vi "Apply force DS345 TDC001 soft tw.vi"(4 "Moving parameters":T2={"Velocity (mm/s)"=0.5, "Abs position (mm)"=0.0, "Lasting time (s)"=20.0}, 5 "Lasting time (s)":dbl=10.0, 6 "TDC001 motor Serial":i32=83858441, 7 "Apply force":bool, 8 "Cluster":T1={"Osc. Amp. (V)"=0.06, "Osc. Freq. (Hz)"=1200.0} {"Osc. Freq. (Hz)" min=0.001 max=250000.0 step=0.001 format="%.3f"; "Osc. Amp. (V)" min=0.0 max=10.0 step=0.001 format="%.3f"}, 9 "Default setting (DS345)":T1={"Osc. Amp. (V)"=0.01, "Osc. Freq. (Hz)"=1000.0} {"Osc. Freq. (Hz)" min=0.001 max=250000.0 step=0.001 format="%.3f"; "Osc. Amp. (V)" min=0.0 max=0.1 step=0.001 format="%.3f"}, 10 "SRS DS345 GPIB address":string="0:18") -> ()   [LabVIEW 2015]
panel:
  out "Working":bool
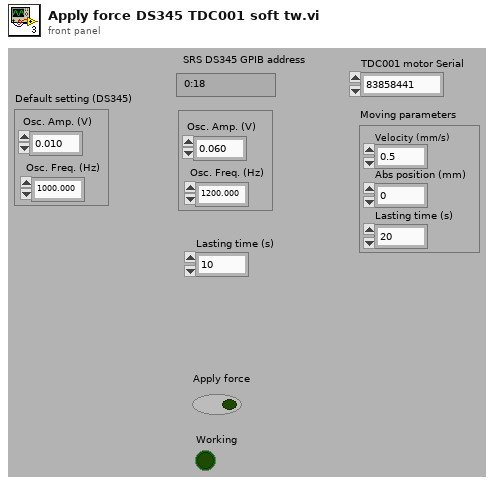
[diagram p1: front panel]
types:
  T1 = cluster{"Osc. Amp. (V)":dbl, "Osc. Freq. (Hz)":dbl}
  T2 = cluster{"Velocity (mm/s)":dbl, "Abs position (mm)":dbl, "Lasting time (s)":dbl}
  T3 = cluster{"Velocity (mm/s)":dbl, dbl, "Lasting time (s)":dbl}
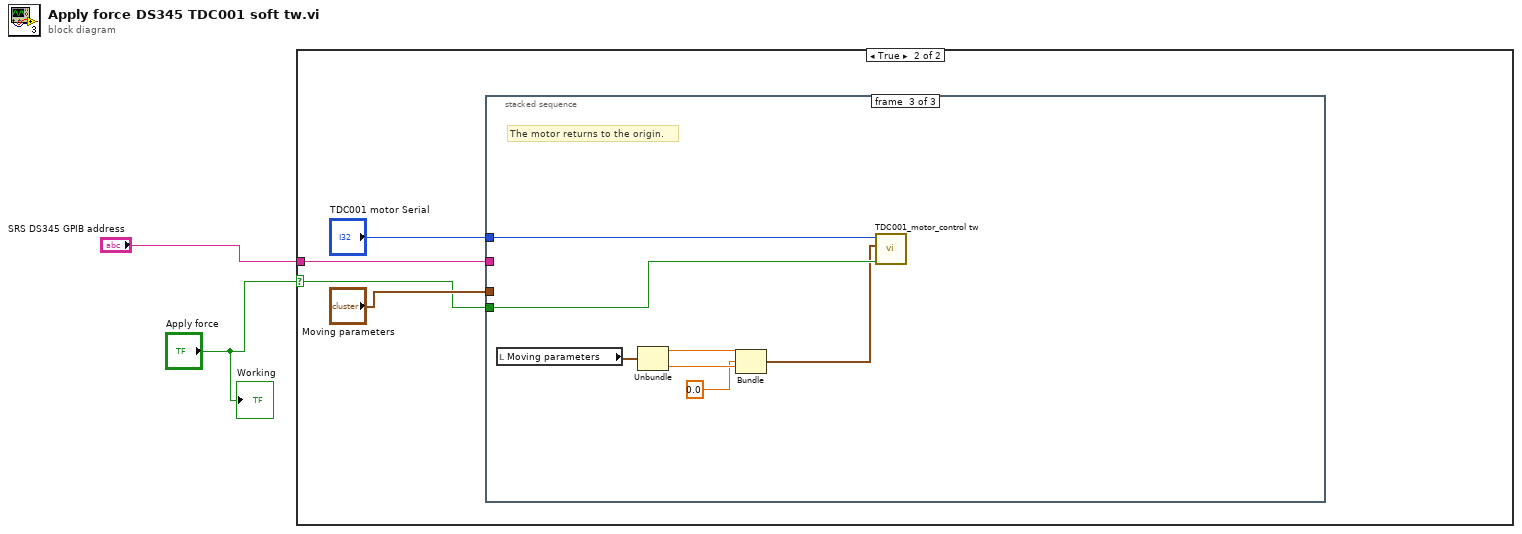
[diagram p0: block diagram]
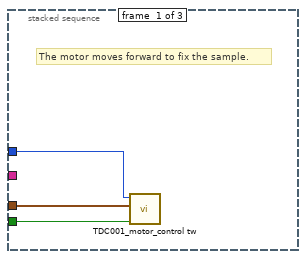
[diagram p3: hidden frame]
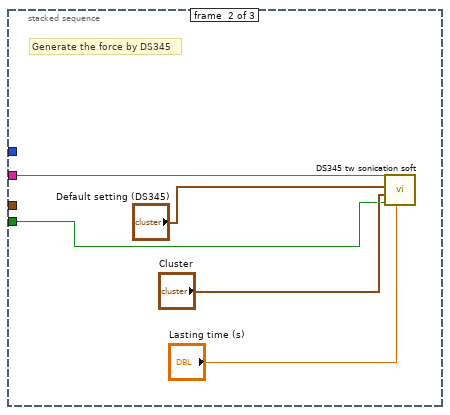
[diagram p4: hidden frame]
diagram:
  n1 = case shown="True" "Apply force" {
    selector: "Apply force" -> [_ w4]
    tunnel: "SRS DS345 GPIB address" -> [_ w3]
    frame False {
    }
    frame True {
      n2 = stacked-sequence {
        tunnel: "TDC001 motor Serial" -> [w9 _ w21]
        tunnel: "Moving parameters" -> [w8 _ _]
        tunnel: w4 -> [w7 w10 w20]
        tunnel: w3 -> [_ w14 _]
        frame #0 {
          # "The motor moves forward to fix the sample."
          n3 = call "TDC001_motor_control tw.vi"("Move"=w7, "Moving parameters"=w8, "Serial"=w9) -> ()  [unwired: 8 in, 1 out]
        }
        frame #1 {
          # "Generate the force by DS345"
          n4 = call "DS345 tw sonication soft.vi"("SRS DS345 GPIB address"=w14, "Default setting (DS345)"="Default setting (DS345)", "Cluster"="Cluster", "Lasting time (s)"="Lasting time (s)", "Apply force"=w10) -> ()  [unwired: 4 in]
        }
        frame #2 {
          # "The motor returns to the origin."
          n5 = local read "Moving parameters"() -> (w19:T2)
          n6 = Unbundle(w19) -> ("Velocity (mm/s)"=w18:dbl, "Lasting time (s)"=w17:dbl)  [unwired: 1 out]
          n7 = Bundle("Velocity (mm/s)"=w18, 0.0, "Lasting time (s)"=w17) -> (w15:T3)  [unwired: 1 in]
          n8 = call "TDC001_motor_control tw.vi"("Move"=w20, "Moving parameters"=w15, "Serial"=w21) -> ()  [unwired: 8 in, 1 out]
        }
      }
    }
  }
  "Working" <- "Apply force"
